vi "Vector Cross Product.vi"(2 "B":dbl[](array[numeric]), 3 "A":dbl[](array[numeric])) -> (1 "A x B":dbl[](array[numeric]))   [LabVIEW 2024]
panel:
  # "i  j  k\n 1  2  3\n 2  1  0"
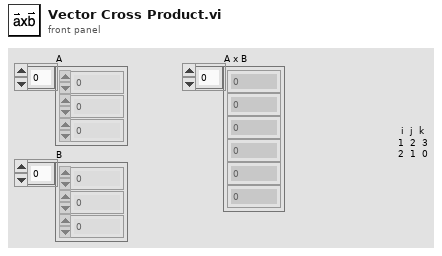
[diagram p1: front panel]
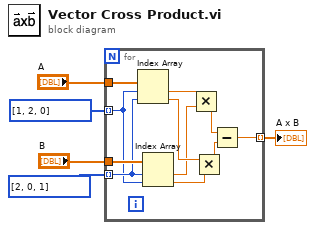
[diagram p0: block diagram]
diagram:
  n1 = for {
    tunnel: "A" -> [w16]
    tunnel: "B" -> [w15]
    tunnel: i32[] [1, 2, 0] -> [w6] mode=indexing
    tunnel: i32[] [2, 0, 1] -> [w7] mode=indexing
    tunnel: [w10] -> w4 mode=indexing
    n2 = Index Array(array=w16, index #1=w6, index #2=w7) -> (element #1=w14:dbl, element #2=w13:dbl)
    n3 = Index Array(array=w15, index #1=w7, index #2=w6) -> (element #1=w9:dbl, element #2=w8:dbl)
    n4 = Multiply(x=w14, y=w9) -> (x*y=w11:dbl)
    n5 = Multiply(x=w13, y=w8) -> (x*y=w12:dbl)
    n6 = Subtract(x=w11, y=w12) -> (x-y=w10:dbl)
  }
  "A x B" <- w4
